vi "Special Write.vi"(8 "error in (no error)":errorcluster, 10 "Input String":string, 11 "VISA resource name":refnum<visa-resource-name>) -> (0 "error out":errorcluster, 3 "VISA resource name out":refnum<visa-resource-name>)   [LabVIEW 2015, in "Ohaus AV Series.lvlib"]
doc: "This VI uses a VISA Write to write individual characters of the command string to the balance. It also writes a carriage return (\\r) as a termination character."
uses:
  Ohaus AV Series.lvlib
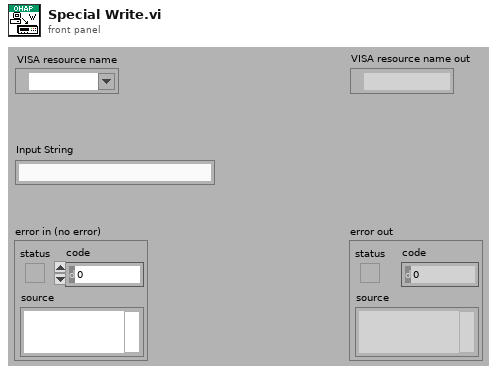
[diagram p1: front panel]
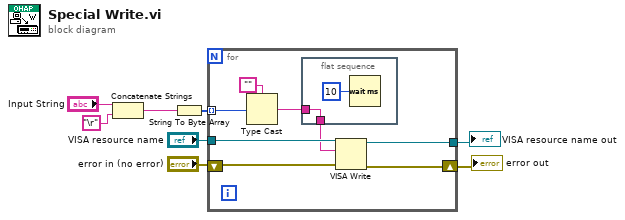
[diagram p0: block diagram]
diagram:
  n1 = Concatenate Strings("Input String", "\r") -> (w6:string)
  n2 = String To Byte Array(string=w6) -> (unsigned byte array=w5:u8[])
  n3 = for {
    tunnel: w5 -> [w11] mode=indexing
    tunnel: [w16] -> w4
    tunnel: "VISA resource name" -> [w14]
    shift-right: [w15] -> w3
    shift-left: "error in (no error)" -> [w13]
    n4 = Type Cast(type="", x=w11) -> (*(type *) &x=w10:string)
    n5 = flat-sequence {
      tunnel: w10 -> [w17]
      tunnel: [w17] -> w9
      frame #0 {
        n6 = Wait (ms)(milliseconds to wait=u32 10) -> ()  [unwired: 1 out]
      }
    }
    n7 = VISA Write(VISA resource name=w14, write buffer=w9, error in (no error)=w13) -> (VISA resource name out=w16:refnum<visa-resource-name>, error out=w15:errorcluster)  [unwired: 1 out]
  }
  "VISA resource name out" <- w4
  "error out" <- w3
